vi "String to Number Array.vi"(11 "Input String":string) -> (3 "Array":i32[](array[numeric]))   [LabVIEW 2014]
doc: "Converts the string to a 1D numeric array. space = 0, a = 1, b = 2, ... z = 26. And abandon the other characters."
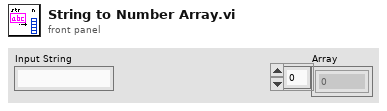
[diagram p1: front panel]
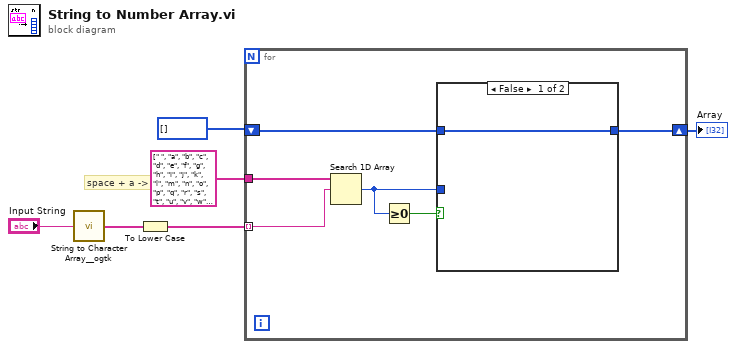
[diagram p0: block diagram]
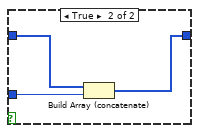
[diagram p2: hidden frame]
diagram:
  # "space + a -> z"
  n1 = call <userlib>:"String to Character Array__ogtk.vi"("Input String"="Input String") -> ("Character Array"=w6:string[])
  n2 = To Lower Case(string=w6) -> (all lower case string=w5:string[])
  n3 = for {
    tunnel: w5 -> [w11] mode=indexing
    tunnel: string[] [" ", "a", "b", "c", "d", "e", "f", "g", "h", "i", "j", "k", "l", "m", "n", "o", "p", "q", "r", "s", "t", "u", "v", "w", "x", "y", "z"] -> [w12]
    shift-right: [w8] -> w2
    shift-left: i32[] [] -> [w7]
    n4 = Search 1D Array(1D array=w12, element=w11) -> (index of element=w9:i32)  [unwired: 1 in]
    n5 = Greater Or Equal To 0?(x=w9) -> (x >= 0?=w10:bool)
    n6 = case shown="False" w10 {
      tunnel: w9 -> [_ w16]
      tunnel: [w13 w15] -> w8
      tunnel: w7 -> [w13 w14]
      frame False {
      }
      frame True {
        n7 = Build Array (concatenate)(w14, w16) -> (w15:i32[])
      }
    }
  }
  "Array" <- w2
